vi "LSX Create LSID.vi"(8 "error in (no error)":errorcluster, 11 "plLSID":i32) -> (0 "error out":errorcluster, 2 "function return":i32, 3 "plLSID out":i32)   [LabVIEW 2018, in "Tango.lvlib"]
doc: "TANGOAPI int TANGOCALL LSX_CreateLSID (int *plLSID);"
uses:
  Tango.lvlib
  SubVIs/Tango_DLL.dll
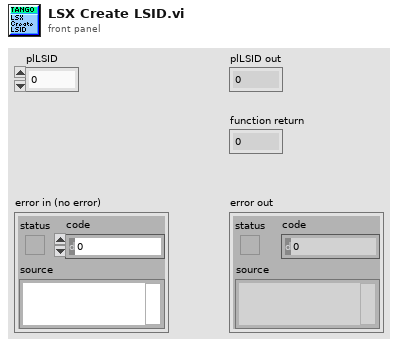
[diagram p1: front panel]
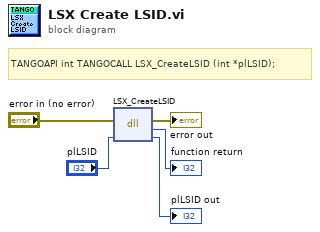
[diagram p0: block diagram]
diagram:
  # "TANGOAPI int TANGOCALL LSX_CreateLSID (int *plLSID);"
  n1 = dll-call lib="C:/Users/Familie/Documents/LabviewIX81/lib/TANGO Stage/SubVIs/Tango_DLL.*" fn="LSX_CreateLSID"(error in="error in (no error)", "plLSID"="plLSID") -> (error out=→"error out":errorcluster, →"function return":i32, "plLSID"=→"plLSID out":i32)  [unwired: 2 in, 1 out]
